vi "获取电脑分辨率.vi"() -> (2 "宽":i32, 3 "长":i32, 4 "子面板路径":string)   [LabVIEW 2015]
uses:
  user32.dll
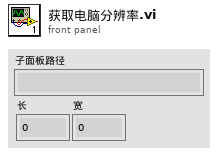
[diagram p1: front panel]
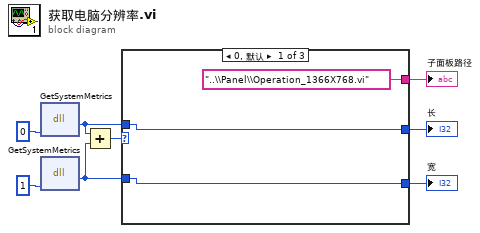
[diagram p0: block diagram]
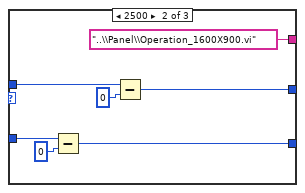
[diagram p2: hidden frame]
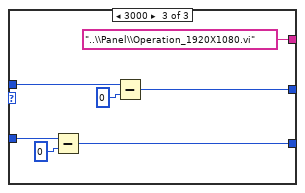
[diagram p3: hidden frame]
diagram:
  n1 = dll-call lib="User32.dll" fn="GetSystemMetrics"("nIndex"=0) -> ("返回类型"=w4:i32)  [unwired: 4 in, 2 out]
  n2 = dll-call lib="User32.dll" fn="GetSystemMetrics"("nIndex"=1) -> ("返回类型"=w2:i32)  [unwired: 4 in, 2 out]
  n3 = Add(x=w4, y=w2) -> (x+y=w6:i32)
  n4 = case shown="0, 默认" w6 {
    tunnel: ["..\\Panel\\Operation_1366X768.vi" ("名称或相对路径") "..\\Panel\\Operation_1600X900.vi" ("名称或相对路径") "..\\Panel\\Operation_1920X1080.vi" ("名称或相对路径")] -> w5
    tunnel: w4 -> [w10 w16 w23]
    tunnel: [w10 w15 w22] -> w3
    tunnel: w2 -> [w9 w13 w20]
    tunnel: [w9 w12 w19] -> w1
    frame 0, Default {
    }
    frame 2500 {
      n5 = Subtract(x=w13, y=0) -> (x-y=w12:i32)
      n6 = Subtract(x=w16, y=0) -> (x-y=w15:i32)
    }
    frame 3000 {
      n7 = Subtract(x=w20, y=0) -> (x-y=w19:i32)
      n8 = Subtract(x=w23, y=0) -> (x-y=w22:i32)
    }
  }
  "子面板路径" <- w5
  "长" <- w3
  "宽" <- w1
